vi "PWM Wing Duty Cycle Calculation.vi"(9 "End Angle Duty Cycle":fxp<+,8,0>, 10 "Start Angle Duty Cycle":fxp<+,8,0>, 11 "Sector":u8) -> (3 "Duty Cycle Out":fxp<+,8,0>)   [LabVIEW 2013]
uses:
  <vilib>/rvi/Analysis/common/FxpNativeNode/niFpgaFxpNative.xnode
  Globals/Sector Parameter Global.vi
panel:
  in  "Previous Sector":i16
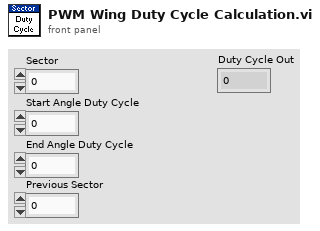
[diagram p1: front panel]
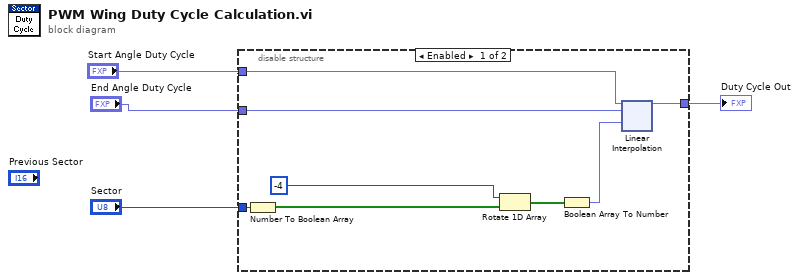
[diagram p0: block diagram]
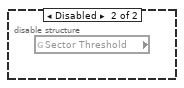
[diagram p2: hidden frame]
diagram:
  n1 = disable-structure shown="Enabled" {
    disable-tunnel: "Start Angle Duty Cycle" -> [w12 _]
    disable-tunnel: "End Angle Duty Cycle" -> [w11 _]
    disable-tunnel: [w10 _] -> w2
    disable-tunnel: "Sector" -> [w9 _]
    frame Enabled {
      n2 = Number To Boolean Array(number=w9) -> (Boolean array=w8:bool[])
      n3 = Rotate 1D Array(1:w8, 2:-4 ("n")) -> (0:w7:bool[])
      n4 = Boolean Array To Number(Boolean array=w7) -> (number=w6:fxp<+,8,0>)
      n5 = xnode ("Linear Interpolation")("y0"=w12, "y1"=w11, "x"=w6) -> ("y"=w10:fxp<+/-,9,1>)
    }
    frame Disabled {
      n6 = global read "Sector Parameter Global.vi" "Sector Threshold"() -> ()  [unwired: 1 out]
    }
  }
  "Duty Cycle Out" <- w2
